vi "Wheel_Normalize.vi"(6 "Max Speed":dbl, 9 "Right Wheel Demand":dbl, 11 "Left Wheel Demand":dbl) -> (1 "Normalized Right Wheel Demand":dbl, 3 "Normalized Left Wheel Demand":dbl)   [LabVIEW 2019, in "PathExecution_Library.lvlib"]
uses:
  PathExecution_Library.lvlib
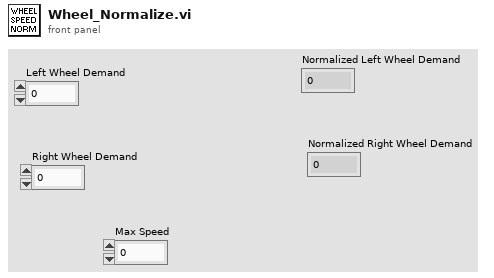
[diagram p1: front panel]
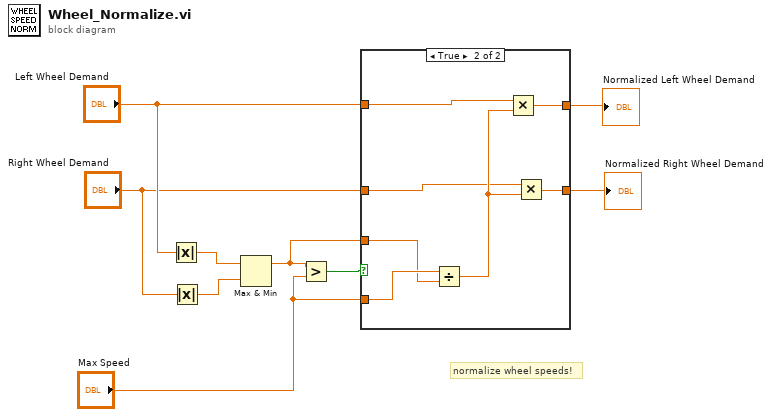
[diagram p0: block diagram]
diagram:
  # "normalize wheel speeds!"
  n1 = Absolute Value(x="Left Wheel Demand") -> (abs(x)=w9:dbl)
  n2 = Absolute Value(x="Right Wheel Demand") -> (abs(x)=w8:dbl)
  n3 = Max & Min(x=w9, y=w8) -> (max(x,y)=w2:dbl)  [unwired: 1 out]
  n4 = Greater?(x=w2, y="Max Speed") -> (0:w1:bool)
  n5 = case shown="True" w1 {
    tunnel: [w11 w14] -> w5
    tunnel: "Left Wheel Demand" -> [w11 w13]
    tunnel: "Right Wheel Demand" -> [w10 w12]
    tunnel: [w10 w15] -> w4
    tunnel: "Max Speed" -> [_ w18]
    tunnel: w2 -> [_ w17]
    frame False {
    }
    frame True {
      n6 = Divide(x=w18, y=w17) -> (x/y=w16:dbl)
      n7 = Multiply(x=w13, y=w16) -> (x*y=w14:dbl)
      n8 = Multiply(x=w12, y=w16) -> (x*y=w15:dbl)
    }
  }
  "Normalized Left Wheel Demand" <- w5
  "Normalized Right Wheel Demand" <- w4
